vi "Generate Time Series.vi"() -> (3 "Time Series":dbl[](graph))   [LabVIEW 2014]
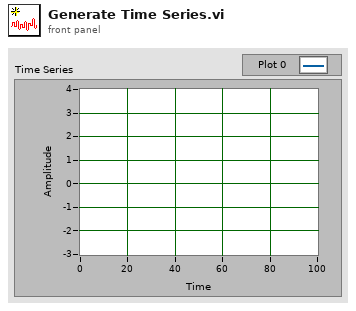
[diagram p1: front panel]
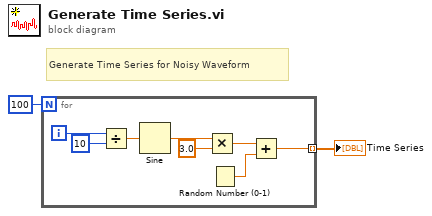
[diagram p0: block diagram]
diagram:
  # "Generate Time Series for Noisy Waveform"
  n1 = for "Generate Time Series for Noisy Waveform" {
    N: 100 -> [_]
    tunnel: [w3] -> w1 mode=indexing
    i -> [w10]
    n2 = Divide(x=w10, y=10) -> (x/y=w9:dbl)
    n3 = Sine(x=w9) -> (sin(x)=w7:dbl)
    n4 = Multiply(x=w7, y=3.0) -> (x*y=w5:dbl)
    n5 = Random Number (0-1)() -> (number: 0 to 1=w4:dbl)
    n6 = Add(x=w5, y=w4) -> (x+y=w3:dbl)
  }
  "Time Series" <- w1
